vi "Tube and DDA Holders.vi"(8 "error in (no error)":errorcluster) -> (0 "error out":errorcluster, 3 "SceneObject out":refnum<vi>)   [LabVIEW 2026, in "XRay CArm.lvclass"]
uses:
  XRay CArm.lvclass
  <vilib>/picture/3D Picture Control/Object/Create Object (drawable).vi
  <vilib>/picture/3D Picture Control/Object/Add Object (reference).vi
  <vilib>/picture/3D Picture Control/NI_3D Picture Control.lvlib
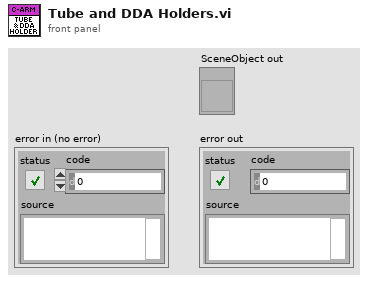
[diagram p1: front panel]
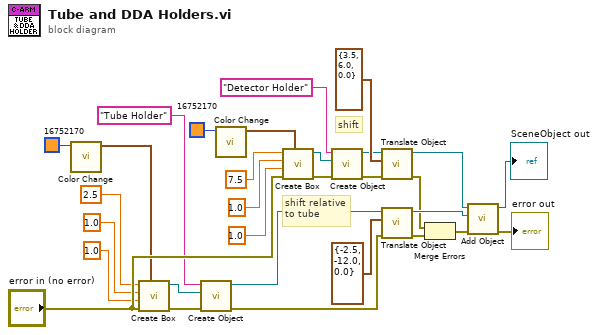
[diagram p0: block diagram]
diagram:
  # "shift relative\nto tube"
  # "shift"
  n1 = call <vilib>:"Color Change.vi"("Color"=u32 16752170) -> ("RGBA"=w17:cluster{"R":sgl, "G":sgl, "B":sgl, "A":sgl})  [unwired: 10 in]
  n2 = call <vilib>:"Create Box.vi"("Color"=w17, "error in (no error)"="error in (no error)", "Length Z"=sgl 1.0 ("Box Length Z"), "Length Y"=sgl 1.0 ("Box Length Y"), "Length X"=sgl 2.5 ("Box Length X")) -> ("error out"=w16:errorcluster, "New Box Refnum"=w15:refnum<vi>)  [unwired: 5 in]
  n3 = call-poly <vilib>:"Create Object.vi"("error in (no error)"=w16, "Geometry"=w15, "Name"="Tube Holder") -> ("error out"=w22:errorcluster, "Scene:New Object"=w14:refnum<vi>)  [unwired: 7 in]
  n4 = call <vilib>:"Color Change.vi"("Color"=u32 16752170) -> ("RGBA"=w2:cluster{"R":sgl, "G":sgl, "B":sgl, "A":sgl})  [unwired: 10 in]
  n5 = call <vilib>:"Create Box.vi"("Color"=w2, "error in (no error)"="error in (no error)", "Length Z"=sgl 1.0 ("Box Length Z"), "Length Y"=sgl 1.0 ("Box Length Y"), "Length X"=sgl 7.5 ("Box Length X")) -> ("error out"=w3:errorcluster, "New Box Refnum"=w4:refnum<vi>)  [unwired: 5 in]
  n6 = call-poly <vilib>:"Create Object.vi"("error in (no error)"=w3, "Geometry"=w4, "Name"="Detector Holder") -> ("error out"=w21:errorcluster, "Scene:New Object"=w5:refnum<vi>)  [unwired: 7 in]
  n7 = call <vilib>:"Translate Object.vi"("error in (no error)"=w21, "Translation"=cluster{"X":sgl, "Y":sgl, "Z":sgl} {"X"=3.5, "Y"=6.0, "Z"=0.0} ("Translation 3"), "Scene.Object In"=w5) -> ("error out"=w24:errorcluster, "Scene.Object Out"=w26:refnum<vi>)  [unwired: 7 in]
  n8 = call <vilib>:"Translate Object.vi"("error in (no error)"=w22, "Translation"=cluster{"X":sgl, "Y":sgl, "Z":sgl} {"X"=-2.5, "Y"=-12.0, "Z"=0.0} ("Translation 3"), "Scene.Object In"=w14) -> ("error out"=w25:errorcluster, "Scene.Object Out"=w27:refnum<vi>)  [unwired: 7 in]
  n9 = Merge Errors(w24, w25) -> (w29:errorcluster)
  n10 = call-poly <vilib>:"Add Object.vi"("error in (no error)"=w29, "New Object In"=w27, "Scene Object In"=w26) -> ("error out"=→"error out":errorcluster, "Scene Object Out"=→"SceneObject out":refnum<vi>)  [unwired: 6 in, 1 out]
